vi "Init TDMS Channel.vi"(0 "Group":string, 2 "Interpolation Settings":T2, 5 "Channel":string, 7 "tdms file":refnum<k34>, 9 "Ref in":T1 format="%.0x", 11 "error in (no error)":errorcluster) -> (6 "dt out":dbl, 8 "Samples":u32, 10 "Ref out":T1=18446744073709551615 format="%.0x", 15 "error out":errorcluster)   [LabVIEW 2011, in "TDMS Custom Device.lvlib"]
uses:
  TDMS Custom Device.lvlib
  <vilib>/NI Veristand/Custom Device API/Custom Device Item Ref.ctl
  <vilib>/NI Veristand/Custom Device API/Set Item Property (Double).vi
  <vilib>/NI Veristand/Custom Device API/Set Item Property (Variant).vi
  <vilib>/NI Veristand/Custom Device API/Set Item Property (I32).vi
  <vilib>/NI Veristand/Custom Device API/Custom Device API.lvlib
  <vilib>/NI Veristand/Custom Device API/Set Item Property (String).vi
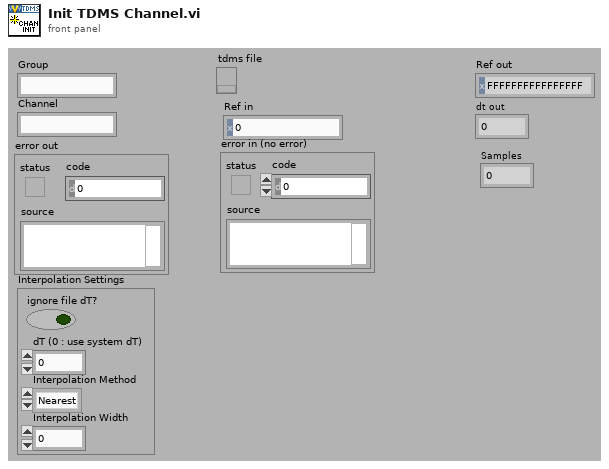
[diagram p1: front panel]
types:
  T1 = typedef "Custom Device API.lvlib/Custom Device Item Ref.ctl" = u64
  T2 = cluster{"ignore file dT?":bool, "dT (0 : use system dT)":dbl, "Interpolation Method ":enum16{"Nearest", "Linear", "Spline", "Cubic Hermite", "Lagrange", "Polynomial"}, "Interpolation Width":i32}
  T3 = cluster{"property name":string, "Property Name":string, enum16{"string", "double", "int"}}[]
  T4 = enum16{"Nearest", "Linear", "Spline", "Cubic Hermite", "Lagrange", "Polynomial"}
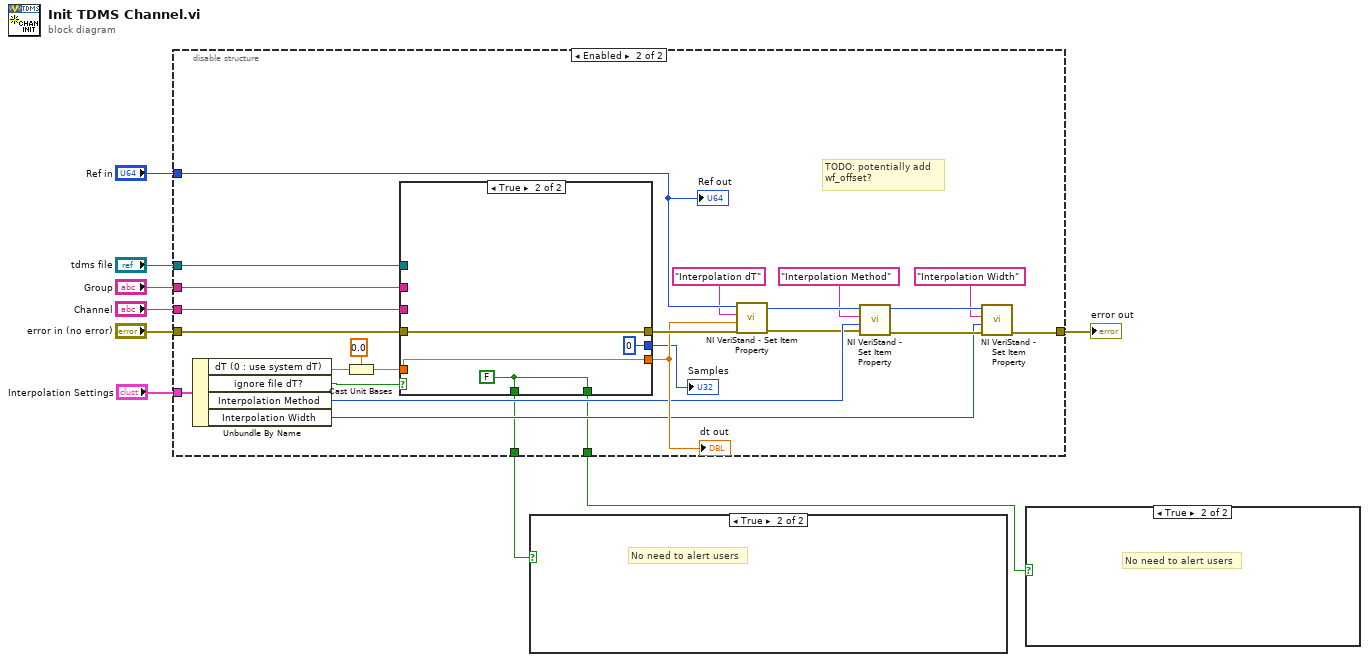
[diagram p0: block diagram]
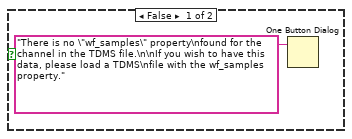
[diagram p2: hidden frame]
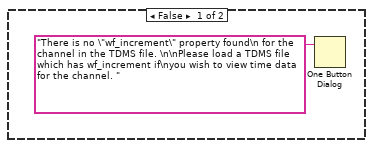
[diagram p3: hidden frame]
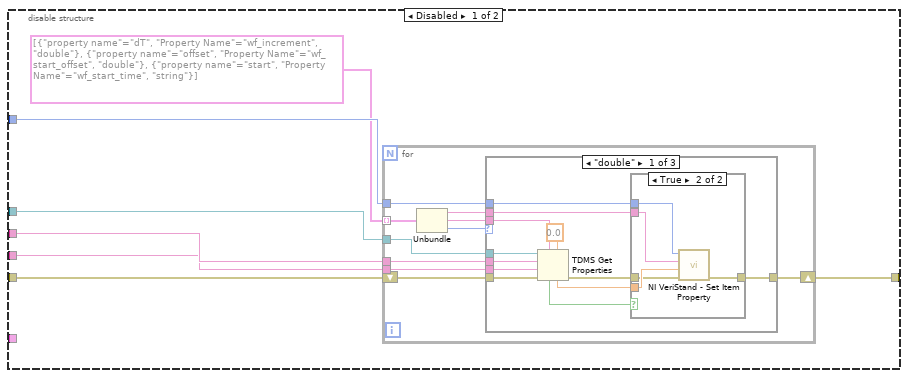
[diagram p4: hidden frame]
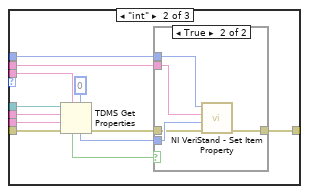
[diagram p6: hidden frame]
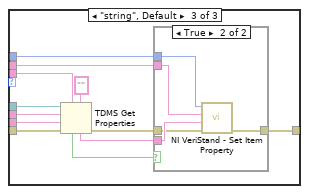
[diagram p8: hidden frame]
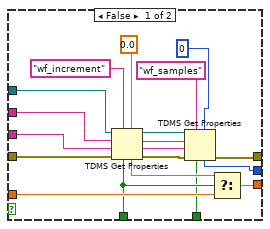
[diagram p10: hidden frame]
diagram:
  n1 = disable-structure shown="Enabled" {
    disable-tunnel: "error in (no error)" -> [w16 w104]
    disable-tunnel: "Group" -> [w15 w103]
    disable-tunnel: "Channel" -> [w14 w102]
    disable-tunnel: "tdms file" -> [w13 w105]
    disable-tunnel: "Ref in" -> [w12 w101]
    disable-tunnel: [w10 w87] -> w4
    disable-tunnel: "Interpolation Settings" -> [_ w100]
    disable-tunnel: [_ w82] -> w2
    disable-tunnel: [_ w81] -> w1
    frame Disabled {
      n2 = for {
        tunnel: w15 -> [w25]
        tunnel: w14 -> [w24]
        tunnel: w13 -> [w23]
        tunnel: w12 -> [w22]
        tunnel: T3 [{"property name"="dT", "Property Name"="wf_increment", enum."double"}, {"property name"="offset", "Property Name"="wf_start_offset", enum."double"}, {"property name"="start", "Property Name"="wf_start_time", enum."string"}] ("output array") -> [w21] mode=indexing
        shift-right: [w20] -> w10
        shift-left: w16 -> [w26]
        n3 = Unbundle(w21) -> ("property name"=w19:string, "Property Name"=w18:string, w17:enum16{"string", "double", "int"})
        n4 = case shown="\"double\"" w17 {
          tunnel: w26 -> [w38 w56 w74]
          tunnel: w25 -> [w37 w55 w73]
          tunnel: w24 -> [w36 w54 w72]
          tunnel: w23 -> [w35 w53 w71]
          tunnel: w22 -> [w34 w52 w70]
          tunnel: [w30 w48 w66] -> w20
          tunnel: w19 -> [w29 w47 w65]
          tunnel: w18 -> [w28 w46 w64]
          frame "double" {
            n5 = TDMS Get Properties(5:0.0, 7:w28, 8:w38, 9:w36, 10:w37, 11:w35) -> (0:w32:errorcluster, 4:w33:dbl, 6:w31:bool)  [unwired: 3 out]
            n6 = case shown="True" w31 {
              tunnel: w34 -> [_ w44]
              tunnel: w33 -> [_ w43]
              tunnel: w29 -> [_ w42]
              tunnel: w32 -> [w39 w41]
              tunnel: [w39 w40] -> w30
              frame False {
              }
              frame True {
                n7 = call-poly <vilib>:"NI VeriStand - Set Item Property.vi"("error in (no error)"=w41, "Value"=w43, "Property Name"=w42, "Item Ref in"=w44) -> ("error out"=w40:errorcluster)  [unwired: 7 out]
              }
            }
          }
          frame "int" {
            n8 = TDMS Get Properties(5:0, 7:w46, 8:w56, 9:w54, 10:w55, 11:w53) -> (0:w50:errorcluster, 4:w51:i32, 6:w49:bool)  [unwired: 3 out]
            n9 = case shown="True" w49 {
              tunnel: w52 -> [_ w62]
              tunnel: w51 -> [_ w61]
              tunnel: w47 -> [_ w60]
              tunnel: w50 -> [w57 w59]
              tunnel: [w57 w58] -> w48
              frame False {
              }
              frame True {
                n10 = call-poly <vilib>:"NI VeriStand - Set Item Property.vi"("error in (no error)"=w59, "Value"=w61, "Property Name"=w60, "Item Ref in"=w62) -> ("error out"=w58:errorcluster)  [unwired: 7 out]
              }
            }
          }
          frame "string", Default {
            n11 = TDMS Get Properties(5:"" ("Property Name"), 7:w64, 8:w74, 9:w72, 10:w73, 11:w71) -> (0:w68:errorcluster, 4:w69:string, 6:w67:bool)  [unwired: 3 out]
            n12 = case shown="True" w67 {
              tunnel: w70 -> [_ w80]
              tunnel: w69 -> [_ w79]
              tunnel: w65 -> [_ w78]
              tunnel: w68 -> [w75 w77]
              tunnel: [w75 w76] -> w66
              frame False {
              }
              frame True {
                n13 = call-poly <vilib>:"NI VeriStand - Set Item Property.vi"("error in (no error)"=w77, "Value"=w79, "Property Name"=w78, "Item Ref in"=w80) -> ("error out"=w76:errorcluster)  [unwired: 7 out]
              }
            }
          }
        }
      }
    }
    frame Enabled {
      # "TODO: potentially add\nwf_offset?"
      n14 = Unbundle By Name(w100) -> ("dT (0 : use system dT)"=w96:dbl, "ignore file dT?"=w97:bool, "Interpolation Method"=w92:T4, "Interpolation Width"=w86:i32)
      n15 = Cast Unit Bases(0:w96, 1:0.0) -> (2:w94:dbl)
      n16 = case shown="True" w97 {
        tunnel: w105 -> [w124 _]
        tunnel: w104 -> [w123 w128]
        tunnel: w103 -> [w122 _]
        tunnel: w102 -> [w121 _]
        tunnel: [w113 w128] -> w99
        tunnel: [w116 w127] -> w98
        tunnel: w94 -> [w117 w127]
        tunnel: [w108 u32 0] -> w83
        tunnel: [w107 w125] -> w82
        tunnel: [w106 w125] -> w81
        frame False {
          n17 = TDMS Get Properties(5:0.0, 7:"wf_increment" ("Property Name"), 8:w123, 9:w121, 10:w122, 11:w124) -> (0:w115:errorcluster, 1:w111:string, 2:w112:string, 3:w114:refnum<k34>, 4:w118:dbl, 6:w107:bool)
          n18 = TDMS Get Properties(5:u32 0, 7:"wf_samples" ("property name"), 8:w115, 9:w111, 10:w112, 11:w114) -> (0:w113:errorcluster, 4:w108:u32, 6:w106:bool)  [unwired: 3 out]
          n19 = Select(t=w118, s=w107, f=w117) -> (s? t:f=w116:dbl)
        }
        frame True {
          w125 = FALSE
        }
      }
      "dt out" <- w98
      "Samples" <- w83
      n20 = call-poly <vilib>:"NI VeriStand - Set Item Property.vi"("error in (no error)"=w99, "Value"=w98, "Property Name"="Interpolation dT", "Item Ref in"=w101) -> ("error out"=w90:errorcluster, "Item Ref out"=w91:T1)  [unwired: 6 out]
      n21 = call-poly <vilib>:"NI VeriStand - Set Item Property.vi"("error in (no error)"=w90, "Value"=w92, "Property Name"="Interpolation Method", "Item Ref in"=w91) -> ("error out"=w89:errorcluster, "Item Ref out"=w88:T1)  [unwired: 6 out]
      n22 = call-poly <vilib>:"NI VeriStand - Set Item Property.vi"("error in (no error)"=w89, "Value"=w86, "Property Name"="Interpolation Width", "Item Ref in"=w88) -> ("error out"=w87:errorcluster)  [unwired: 7 out]
      "Ref out" <- w101
    }
  }
  "error out" <- w4
  n23 = case shown="True" w2 {
    frame False {
      n24 = One Button Dialog(message="There is no \"wf_increment\" property found\n for the channel in the TDMS file. \n\nPlease load a TDMS file which has wf_increment if\nyou wish to view time data for the channel. ") -> ()  [unwired: 1 in, 1 out]
    }
    frame True {
      # "No need to alert users"
    }
  }
  n25 = case shown="True" w1 {
    frame False {
      n26 = One Button Dialog(message="There is no \"wf_samples\" property\nfound for the channel in the TDMS file.\n\nIf you wish to have this data, please load a TDMS\nfile with the wf_samples property.") -> ()  [unwired: 1 in, 1 out]
    }
    frame True {
      # "No need to alert users"
    }
  }
